vi "HEWH Find Vn.vi"(8 "error in (no error)":errorcluster, 11 "UEF Calculated Values Input":T1 {"Data Indexes"."15 sec after Draw Index" format="%#.2f"; "Data Indexes"."15 sec after Draw Timestamp" format="%#.2f"; "Data Indexes"."Test Start Timestamp" format="%.2f"; "Data Indexes"."Test End Timestamp" format="%.2f"; "Data Indexes"."T0 Timestamp" format="%.2f"; "Data Indexes"."Tsf Timestamp" format="%.2f"; "Data Indexes"."Tsu0 Timestamp" format="%.2f"; "Data Indexes"."Tmax1 Timestamp" format="%.2f"; "Data Indexes"."Draw Index Timestamp" format="%#.2f"; "Data Indexes"."Non-Draw Timestamp" format="%#.2f"; "Data Indexes"."Heating Timestamp" format="%#.2f"; "Data Indexes"."Start Energy (BTU-Gas)" format="%.6f"; "Data Indexes"."Start Watt Hours" format="%.6f"; "Static Data"."V - Volume of Wh (True)" format="%.5f"; "Static Data"."T-Ambinet Nominal (°F)" format="%.5f"; "Static Data"."T-Inlet Setpoint (°F)" format="%.5f"; "Static Data"."T-Wh Setpoint (°F)" format="%.5f"; "Sampled Data"."Qe (Wh)" format="%.5f"; "Sampled Data"."Tau stby2 (hr)" format="%.5f"; "Sampled Data"."Tastby2 (°F)" format="%.5f"; "Sampled Data"."Qf (BTU)" format="%.5f"; "Sampled Data"."Qe (BTU)" format="%.5f"; "Sampled Data"."Tmax1 (°F)" format="%.5f"; "Sampled Data"."T0 (°F)" format="%.5f"; "Sampled Data"."Qr (BTU)" format="%.5f"; "Sampled Data"."T 24(°F)" format="%.5f"; "Sampled Data"."T astby(°F)" format="%.5f"; "Sampled Data"."T tstby(°F)" format="%.5f"; "Sampled Data"."T su0(°F)" format="%.5f"; "Sampled Data"."T suf(°F)" format="%.5f"; "Sampled Data"."Tau stby_1 (hr)" format="%.5f"; "Sampled Data"."Qsuf (BTU)" format="%.5f"; "Sampled Data"."Qsu0 (BTU)" format="%.5f"; "Calculated Values"."Draw Bonus Volume (gal)" format="%.6f"; "Calculated Values"."Adjustment Factor" format="%.6f"; "Calculated Values"."T*avg_del(n-1)" format="%.6f"; "Calculated Values"."T*min(n-1)" format="%.6f"; "Calculated Values"."T*avg_del(n)" format="%.6f"; "Calculated Values"."Vn" format="%.6f"; "Calculated Values"."Qdm (BTU)" format="%.6f"; "Calculated Values"."QHWD (BTU)" format="%.6f"; "Calculated Values"."QHW (BTU)" format="%.6f"; "Calculated Values"."UEF" format="%.6f"; "Calculated Values"."QHW67 (BTU)" format="%.6f"; "Calculated Values"."Qda (BTU)" format="%.6f"; "Calculated Values"."Qd (BTU)" format="%.6f"; "Calculated Values"."Q (BTU)" format="%.6f"; "Calculated Values"."UA (BTU/(hr*F))" format="%.6f"; "Calculated Values"."Qhr (BTU/hr)" format="%.6f"; "Calculated Values"."Qstby (BTU)" format="%.6f"; "Calculated Values"."nu_r" format="%.6f"; "Calculated Values"."CpUEF (BTU/(lb*F))" format="%.6f"; "Calculated Values"."rho_nu (lb/gal)" format="%.6f"; "Calculated Values"."V1- Vol (Gal)" format="%.6f"; "Calculated Values"."M cluster mass removed (lb)" format="%.6f"; "Calculated Values"."Cp theoretical (BTU/(lbm °F))" format="%.6f"; "Calculated Values"."Tin1 - Mean Inlet 1st Cluster (°F)" format="%.6f"; "Calculated Values"."Tdel1-Mean Outlet 1st Cluster(°F)" format="%.6f"; "Calculated Values"."Cp 24 (BTU/(lb*F))" format="%.6f"; "Calculated Values"."Cp standby (BTU/(lb*F))" format="%.6f"; "Calculated Values"."Cp2 (BTU/(lb*F))" format="%.6f"; "Calculated Values"."Cp1 (BTU/(lb*F))" format="%.6f"; "Calculated Values"."rho 24 (lb/gal)" format="%.6f"; "Calculated Values"."rho standby (lb/gal)" format="%.6f"; "Calculated Values"."rho 2 (lb/gal)" format="%.6f"; "Calculated Values"."Density of cold water All (lbm/gal)" format="%#.3g"; "Calculated Values"."CpHW (BTU/(lbm °F))" format="%#.3g"; "Calculated Values"."Density of hot water All (lbm/gal)" format="%#.3g"; "Calculated Values"."Mass of water All (lbm)" format="%#.3f"}) -> (0 "error out":errorcluster, 3 "UEF Calculated Values Output":T1 {"Data Indexes"."15 sec after Draw Index" format="%#.2f"; "Data Indexes"."15 sec after Draw Timestamp" format="%#.2f"; "Data Indexes"."Test Start Timestamp" format="%.2f"; "Data Indexes"."Test End Timestamp" format="%.2f"; "Data Indexes"."T0 Timestamp" format="%.2f"; "Data Indexes"."Tsf Timestamp" format="%.2f"; "Data Indexes"."Tsu0 Timestamp" format="%.2f"; "Data Indexes"."Tmax1 Timestamp" format="%.2f"; "Data Indexes"."Draw Index Timestamp" format="%#.2f"; "Data Indexes"."Non-Draw Timestamp" format="%#.2f"; "Data Indexes"."Heating Timestamp" format="%#.2f"; "Data Indexes"."Start Energy (BTU-Gas)" format="%.6f"; "Data Indexes"."Start Watt Hours" format="%.6f"; "Static Data"."V - Volume of Wh (True)" format="%.5f"; "Static Data"."T-Ambinet Nominal (°F)" format="%.5f"; "Static Data"."T-Inlet Setpoint (°F)" format="%.5f"; "Static Data"."T-Wh Setpoint (°F)" format="%.5f"; "Sampled Data"."Qe (Wh)" format="%.5f"; "Sampled Data"."Tau stby2 (hr)" format="%.5f"; "Sampled Data"."Tastby2 (°F)" format="%.5f"; "Sampled Data"."Qf (BTU)" format="%.5f"; "Sampled Data"."Qe (BTU)" format="%.5f"; "Sampled Data"."Tmax1 (°F)" format="%.5f"; "Sampled Data"."T0 (°F)" format="%.5f"; "Sampled Data"."Qr (BTU)" format="%.5f"; "Sampled Data"."T 24(°F)" format="%.5f"; "Sampled Data"."T astby(°F)" format="%.5f"; "Sampled Data"."T tstby(°F)" format="%.5f"; "Sampled Data"."T su0(°F)" format="%.5f"; "Sampled Data"."T suf(°F)" format="%.5f"; "Sampled Data"."Tau stby_1 (hr)" format="%.5f"; "Sampled Data"."Qsuf (BTU)" format="%.5f"; "Sampled Data"."Qsu0 (BTU)" format="%.5f"; "Calculated Values"."Draw Bonus Volume (gal)" format="%.6f"; "Calculated Values"."Adjustment Factor" format="%.6f"; "Calculated Values"."T*avg_del(n-1)" format="%.6f"; "Calculated Values"."T*min(n-1)" format="%.6f"; "Calculated Values"."T*avg_del(n)" format="%.6f"; "Calculated Values"."Vn" format="%.6f"; "Calculated Values"."Qdm (BTU)" format="%.6f"; "Calculated Values"."QHWD (BTU)" format="%.6f"; "Calculated Values"."QHW (BTU)" format="%.6f"; "Calculated Values"."UEF" format="%.6f"; "Calculated Values"."QHW67 (BTU)" format="%.6f"; "Calculated Values"."Qda (BTU)" format="%.6f"; "Calculated Values"."Qd (BTU)" format="%.6f"; "Calculated Values"."Q (BTU)" format="%.6f"; "Calculated Values"."UA (BTU/(hr*F))" format="%.6f"; "Calculated Values"."Qhr (BTU/hr)" format="%.6f"; "Calculated Values"."Qstby (BTU)" format="%.6f"; "Calculated Values"."nu_r" format="%.6f"; "Calculated Values"."CpUEF (BTU/(lb*F))" format="%.6f"; "Calculated Values"."rho_nu (lb/gal)" format="%.6f"; "Calculated Values"."V1- Vol (Gal)" format="%.6f"; "Calculated Values"."M cluster mass removed (lb)" format="%.6f"; "Calculated Values"."Cp theoretical (BTU/(lbm °F))" format="%.6f"; "Calculated Values"."Tin1 - Mean Inlet 1st Cluster (°F)" format="%.6f"; "Calculated Values"."Tdel1-Mean Outlet 1st Cluster(°F)" format="%.6f"; "Calculated Values"."Cp 24 (BTU/(lb*F))" format="%.6f"; "Calculated Values"."Cp standby (BTU/(lb*F))" format="%.6f"; "Calculated Values"."Cp2 (BTU/(lb*F))" format="%.6f"; "Calculated Values"."Cp1 (BTU/(lb*F))" format="%.6f"; "Calculated Values"."rho 24 (lb/gal)" format="%.6f"; "Calculated Values"."rho standby (lb/gal)" format="%.6f"; "Calculated Values"."rho 2 (lb/gal)" format="%.6f"; "Calculated Values"."Density of cold water All (lbm/gal)" format="%#.3g"; "Calculated Values"."CpHW (BTU/(lbm °F))" format="%#.3g"; "Calculated Values"."Density of hot water All (lbm/gal)" format="%#.3g"; "Calculated Values"."Mass of water All (lbm)" format="%#.3f"})   [LabVIEW 2023]
uses:
  Type Definitions/UEF Constants.ctl
  Type Definitions/HEWH Draw Stats.ctl
  Type Definitions/HEWH FHR Draw Type.ctl
  Type Definitions/FHR Bins.ctl
  Type Definitions/HEWH Meter Type.ctl
panel:
  # "FHR"
  # "FHR"
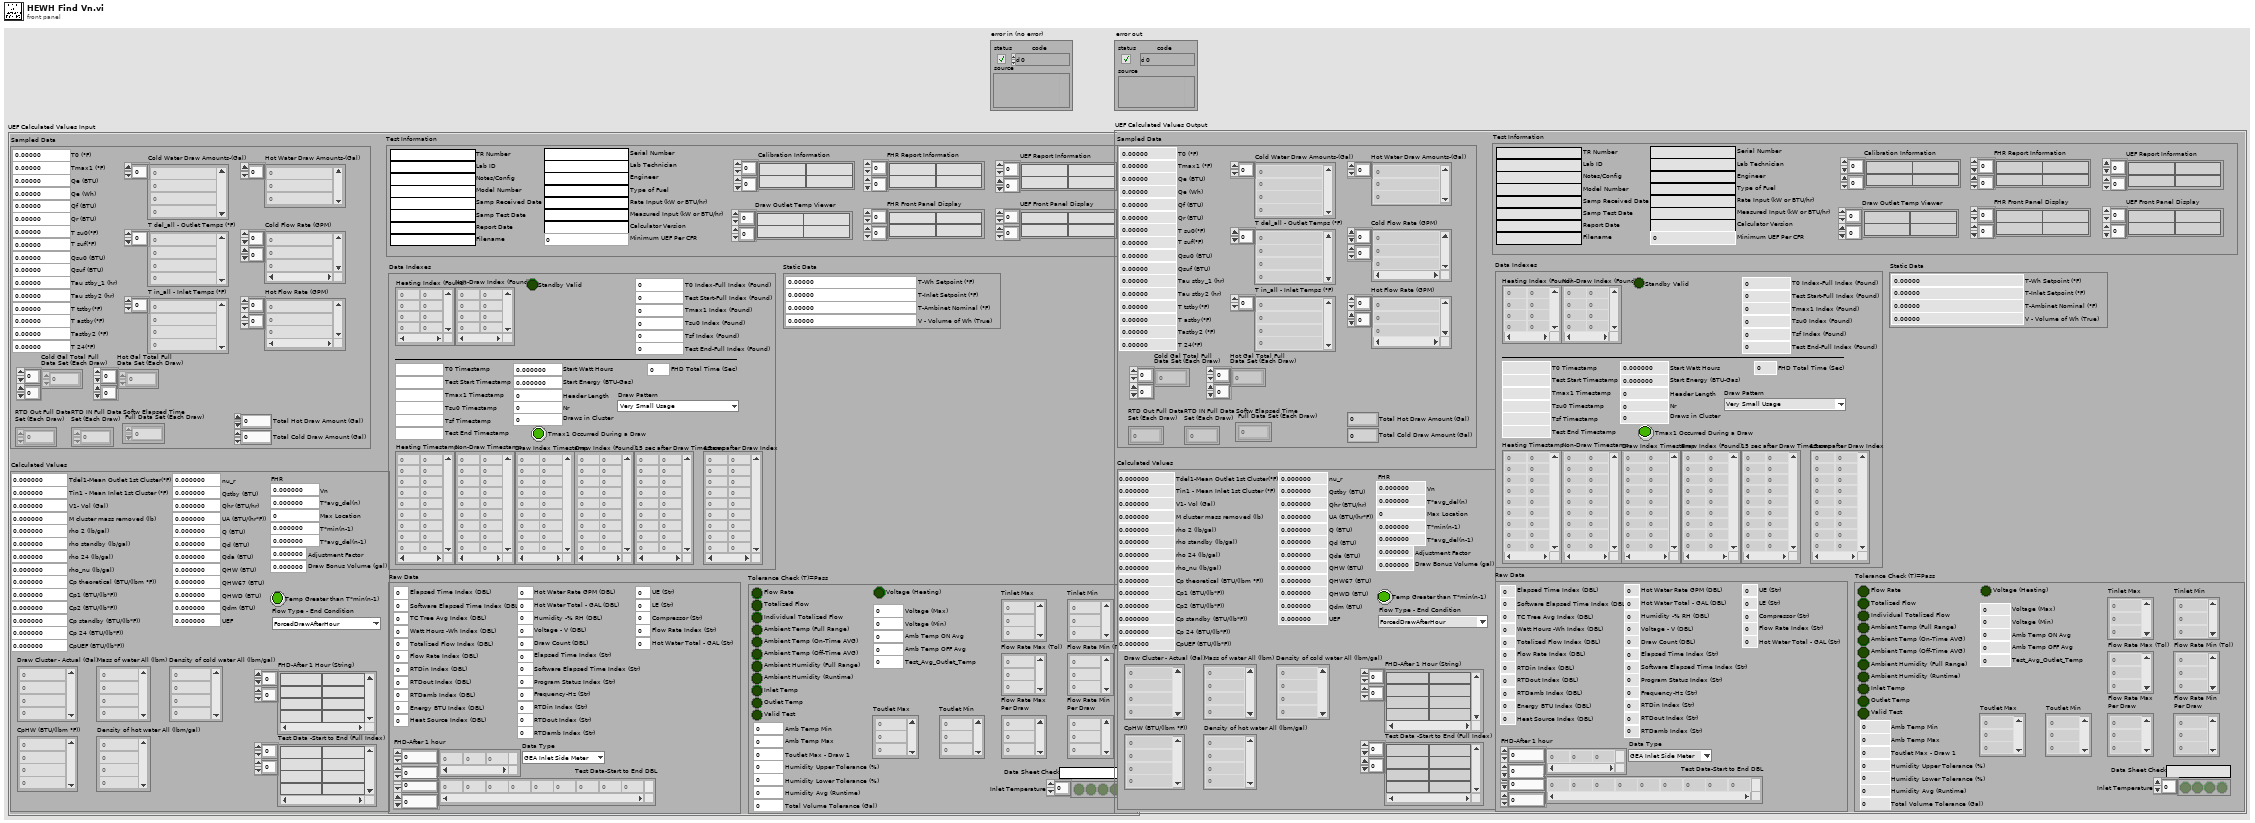
[diagram p1: front panel]
types:
  T1 = typedef "UEF Constants.ctl" = cluster{"Calculated Values":T2, "Sampled Data":cluster{"Cold Water Draw Amounts-(Gal)":dbl[], "T del_all - Outlet Temps (°F)":dbl[], "T in_all - Inlet Temps (°F)":dbl[], "Qsu0 (BTU)":dbl, "Qsuf (BTU)":dbl, "Tau stby_1 (hr)":dbl, "T suf(°F)":dbl, "T su0(°F)":dbl, "T tstby(°F)":dbl, "T astby(°F)":dbl, "T 24(°F)":dbl, "Qr (BTU)":dbl, "T0 (°F)":dbl, "Tmax1 (°F)":dbl, "Qe (BTU)":dbl, "Qf (BTU)":dbl, "Tastby2 (°F)":dbl, "RTD Out Full Data\nSet (Each Draw)":dbl[][], "RTD IN Full Data\nSet (Each Draw)":dbl[][], "Tau stby2 (hr)":dbl, "Hot Water Draw Amounts-(Gal)":dbl[], "Cold Flow Rate (GPM)":dbl[][], "Hot Flow Rate (GPM)":dbl[][], "Softw Elapsed Time\n Full Data Set (Each Draw)":dbl[][], "Cold Gal Total Full\nData Set (Each Draw)":dbl[][], "Total Hot Draw Amount (Gal) ":dbl, "Total Cold Draw Amount (Gal)":dbl, "Qe (Wh)":dbl, "Hot Gal Total Full\nData Set (Each Draw)":dbl[][]}, "Static Data":cluster{"T-Wh Setpoint (°F)":dbl, "T-Inlet Setpoint (°F)":dbl, "T-Ambinet Nominal (°F)":dbl, "V - Volume of Wh (True)":dbl}, "Data Indexes":cluster{"Test Start-Full Index (Found)":i32, "Header Length":i32, "Draw Index (Found)":i32[][], "Nr":i32, "Start Watt Hours":dbl, "Tsu0 Index (Found)":i32, "Tsf Index (Found)":i32, "Start Energy (BTU-Gas)":dbl, "Draws in Cluster":i32, "T0 Index-Full Index (Found)":i32, "Non-Draw Index (Found)":i32[][], "Tmax1 Index (Found)":i32, "Test End-Full Index (Found)":i32, "Heating Index (Found)":i32[][], "Heating Timestamp":dbl[][], "Non-Draw Timestamp":dbl[][], "Draw Index Timestamp":dbl[][], "Tmax1 Timestamp":dbl, "Tsu0 Timestamp":dbl, "Tsf Timestamp":dbl, "T0 Timestamp":dbl, "Test End Timestamp":dbl, "Test Start Timestamp":dbl, "15 sec after Draw Timestamp":dbl[][], "15 sec after Draw Index":dbl[][], "Tmax1 Occurred During a Draw":bool, "FHD Total Time (Sec)":dbl, "Draw Pattern":T4, "Standby Valid":bool}, "Raw Data":cluster{"Elapsed Time Index (DBL)":i32, "Software Elapsed Time Index (DBL)":i32, "TC Tree Avg Index (DBL)":i32, "Watt Hours -Wh Index (DBL)":i32, "Energy BTU Index (DBL)":i32, "Totalized Flow Index (DBL)":i32, "Flow Rate Index (DBL)":i32, "Program Status Index (Str)":i32, "RTDin Index (DBL)":i32, "RTDout Index (DBL)":i32, "RTDamb Index (DBL)":i32, "Test Data-Start to End DBL":dbl[][], "Data Type":T5, "Heat Source Index (DBL)":i32, "Hot Water Rate GPM (DBL)":i32, "Hot Water Total - GAL (DBL)":i32, "FHD-After 1 hour":dbl[][], "Humidity -% RH (DBL)":i32, "Voltage - V (DBL)":i32, "Draw Count (DBL)":i32, "Elapsed Time Index (Str)":i32, "Software Elapsed Time Index (Str)":i32, "Frequency-Hz (Str)":i32, "RTDin Index (Str)":i32, "RTDout Index (Str)":i32, "RTDamb Index (Str)":i32, "UE (Str)":i32, "LE (Str)":i32, "Compressor (Str)":i32, "Flow Rate Index (Str)":i32, "Hot Water Total - GAL (Str)":i32}, "Tolerance Check (T)=Pass":cluster{"Flow Rate":bool, "Totalized Flow":bool, "Ambient Temp (Full Range)":bool, "Ambient Humidity (Full Range)":bool, "Inlet Temp":bool, "Outlet Temp":bool, "Valid Test":bool, "Individual Totalized Flow":bool, "Data Sheet Check":string, "Inlet Temperature":bool[], "Tinlet Max":dbl[], "Tinlet Min":dbl[], "Flow Rate Max (Tol)":dbl[], "Flow Rate Min (Tol)":dbl[], "Amb Temp Max":dbl, "Amb Temp Min":dbl, "Toutlet Max - Draw 1":dbl, "Humidity Upper Tolerance (%)":dbl, "Total Volume Tolerance (Gal)":dbl, "Humidity Lower Tolerance (%)":dbl, "Flow Rate Max\nPer Draw":dbl[], "Flow Rate Min\nPer Draw":dbl[], "Ambient Humidity (Runtime)":bool, "Humidity Avg (Runtime)":dbl, "Ambient Temp (On-Time AVG)":bool, "Ambient Temp (Off-Time AVG)":bool, "Amb Temp OFF Avg":dbl, "Amb Temp ON Avg":dbl, "Voltage (Heating)":bool, "Voltage (Min)":dbl, "Voltage (Max)":dbl, "Toutlet Max":dbl[], "Toutlet Min":dbl[], "Test_Avg_Outlet_Temp":dbl}, "Test Information":cluster{"TR Number":string, "Lab ID":string, "Notes/Config":string, "Model Number":string, "Serial Number":string, "Lab Technician":string, "Engineer":string, "Type of Fuel":string, "Samp Received Date":string, "Samp Test Date":string, "Report Date":string, "Rate Input (kW or BTU/hr)":string, "Measured Input (kW or BTU/hr)":string, "Filename":string, "Calibration Information":string[][], "Calculator Version":string, "Minimum UEF Per CFR":dbl, "UEF Report Information":string[][], "FHR Report Information":string[][], "FHR Front Panel Display":string[][], "UEF Front Panel Display":string[][], "Draw Outlet Temp Viewer":string[][]}}
  T2 = typedef "HEWH Draw Stats.ctl" = cluster{"Draw Cluster - Actual (Gal)":dbl[], "Mass of water All (lbm)":dbl[], "Density of hot water All (lbm/gal)":dbl[], "CpHW (BTU/(lbm °F))":dbl[], "rho 2 (lb/gal)":dbl, "rho standby (lb/gal)":dbl, "rho 24 (lb/gal)":dbl, "Cp1 (BTU/(lb*F))":dbl, "Cp2 (BTU/(lb*F))":dbl, "Cp standby (BTU/(lb*F))":dbl, "Cp 24 (BTU/(lb*F))":dbl, "nu_r":dbl, "Qstby (BTU)":dbl, "Qhr (BTU/hr)":dbl, "UA (BTU/(hr*F))":dbl, "Q (BTU)":dbl, "Qd (BTU)":dbl, "Qda (BTU)":dbl, "QHW67 (BTU)":dbl, "UEF":dbl, "Tdel1-Mean Outlet 1st Cluster(°F)":dbl, "Tin1 - Mean Inlet 1st Cluster (°F)":dbl, "Cp theoretical (BTU/(lbm °F))":dbl, "M cluster mass removed (lb)":dbl, "V1- Vol (Gal)":dbl, "Test Data -Start to End (Full Index)":string[][], "rho_nu (lb/gal)":dbl, "Density of cold water All (lbm/gal)":dbl[], "CpUEF (BTU/(lb*F))":dbl, "QHW (BTU)":dbl, "QHWD (BTU)":dbl, "Qdm (BTU)":dbl, "FHD-After 1 Hour (String)":string[][], "Vn":dbl, "T*avg_del(n)":dbl, "Max Location":i32, "T*min(n-1)":dbl, "T*avg_del(n-1)":dbl, "Temp Greater than T*min(n-1)":bool, "Adjustment Factor":dbl, "Draw Bonus Volume (gal)":dbl, "Flow Type - End Condition":T3}
  T3 = typedef "HEWH FHR Draw Type.ctl" = enum16{"ForcedDrawAfterHour", "HeatingCutoffBeforeHour"}
  T4 = typedef "FHR Bins.ctl" = enum16{"Very Small Usage", "Low Usage", "Medium Usage", "High Usage", "Undefined"}
  T5 = typedef "HEWH Meter Type.ctl" = enum16{"GEA Inlet Side Meter", "GEA Outlet Side Meter", "CSA Inlet Side Meter"}
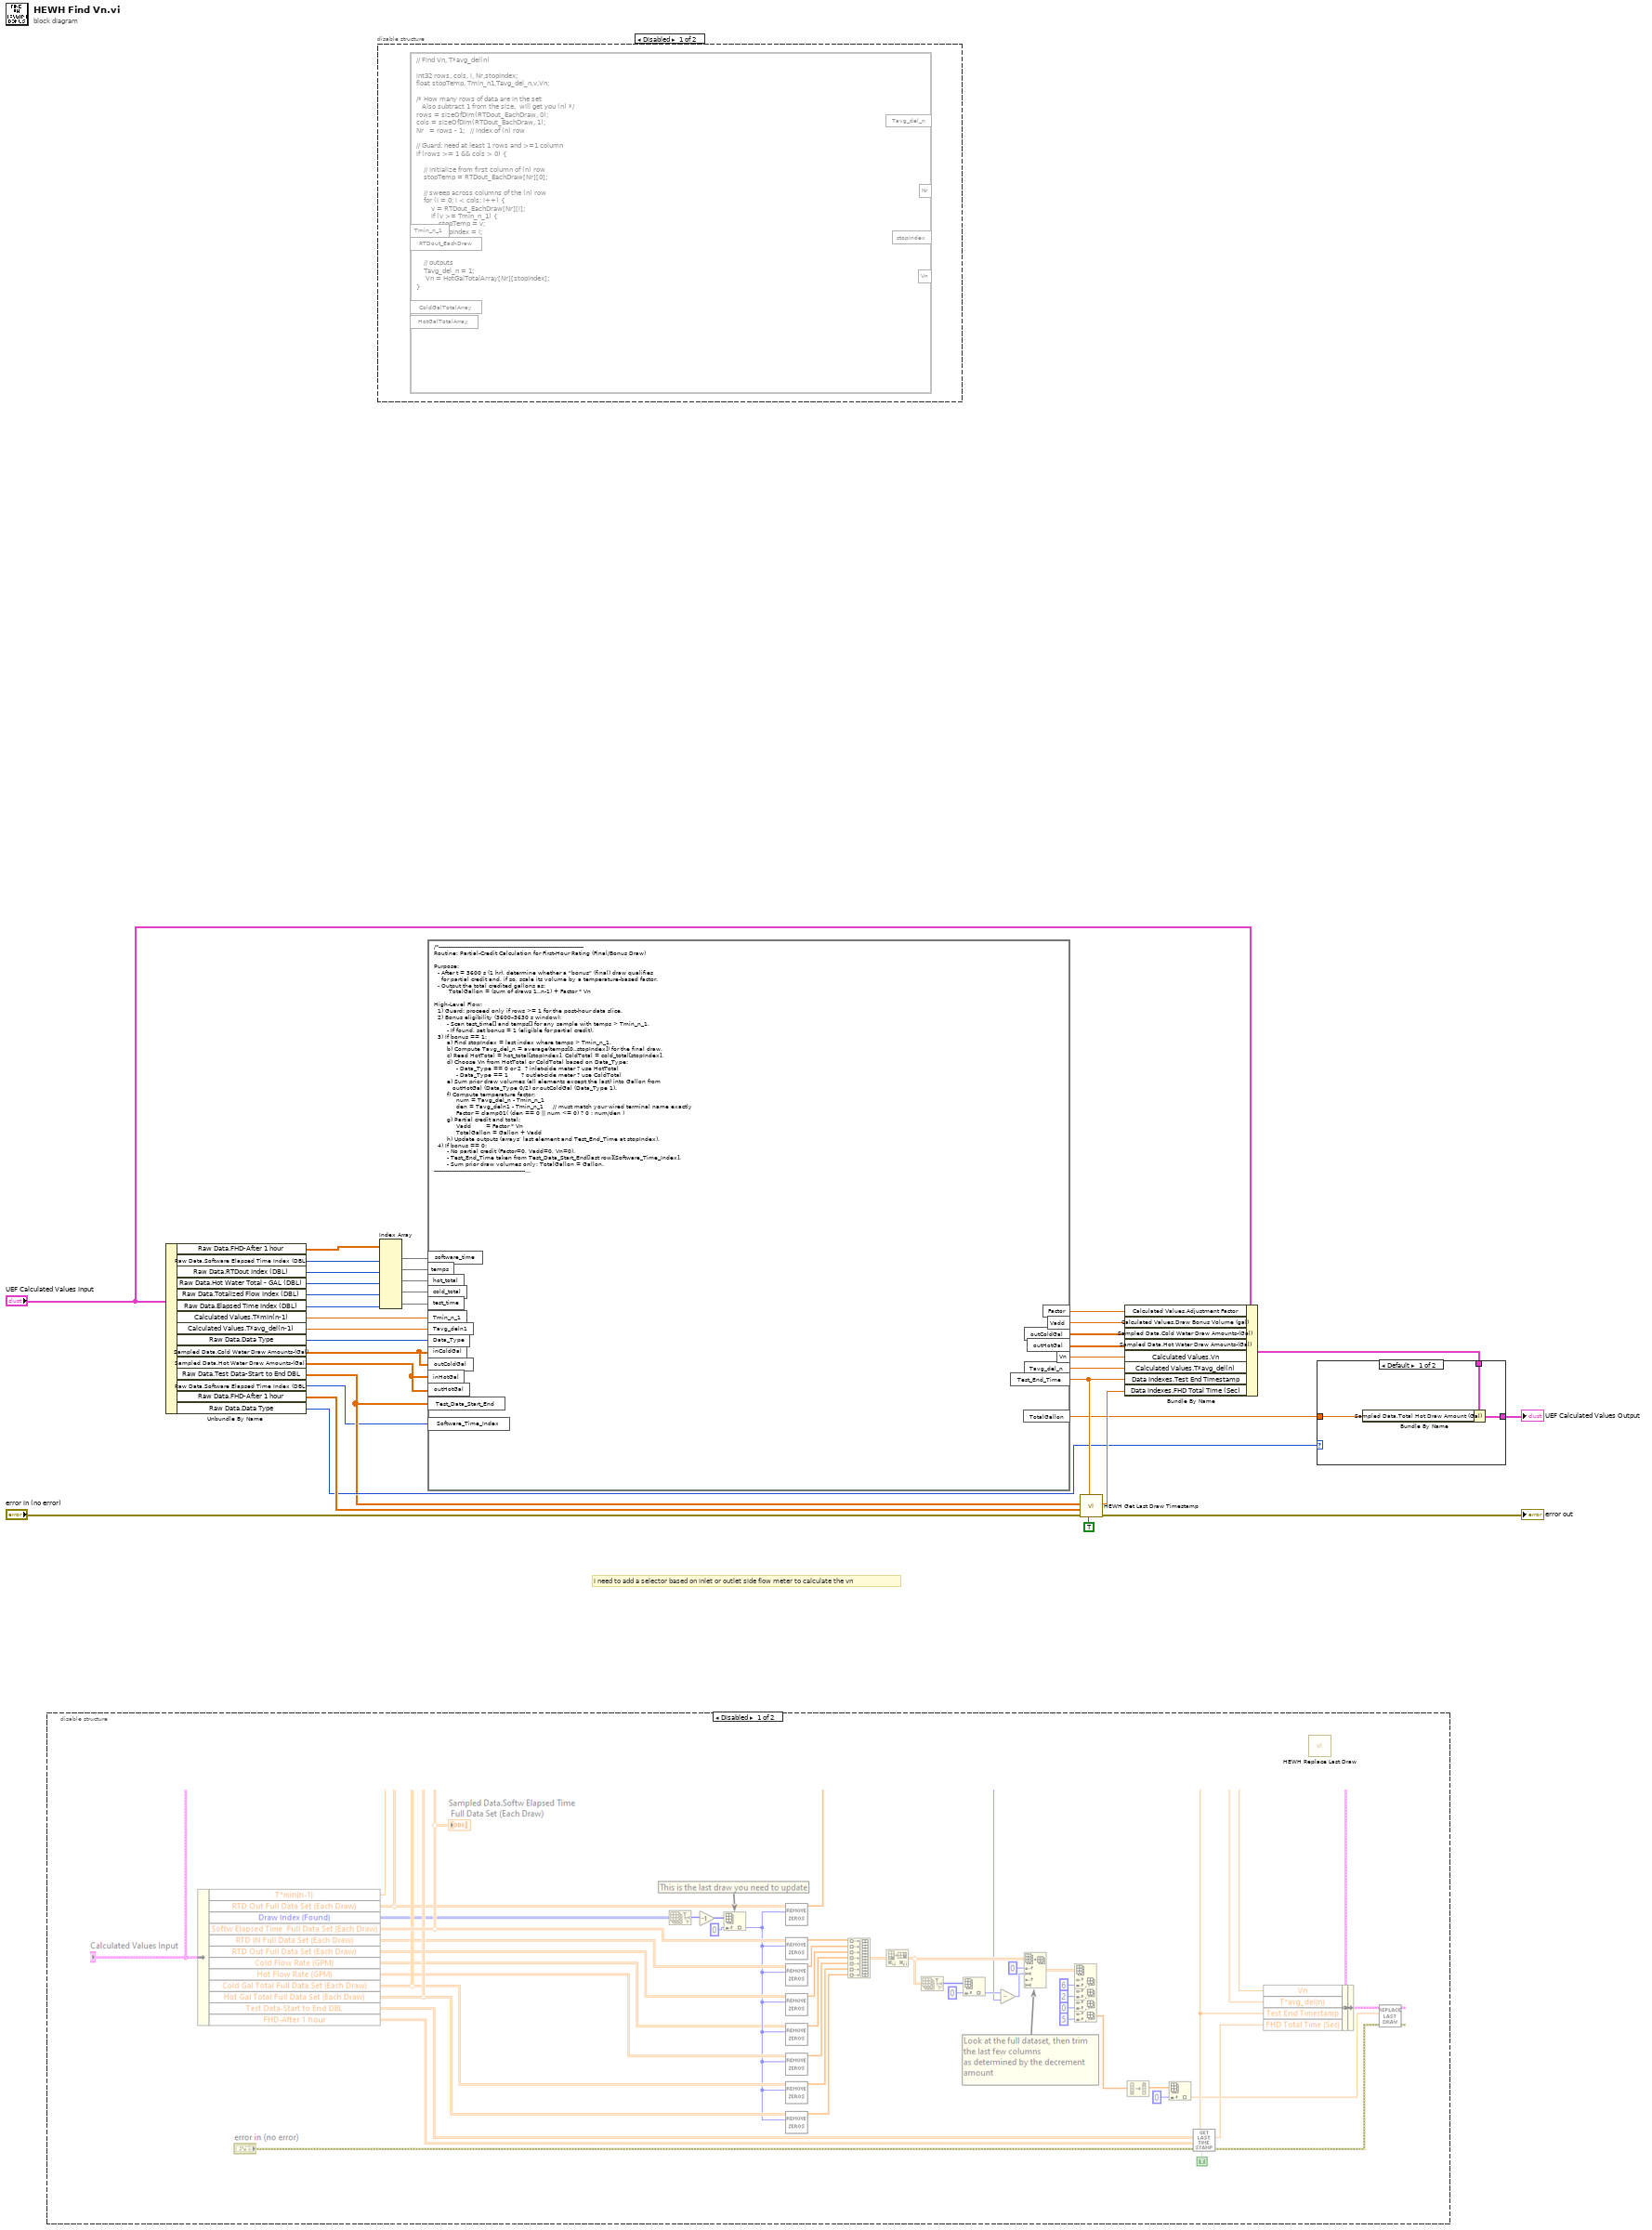
[diagram p0: block diagram]
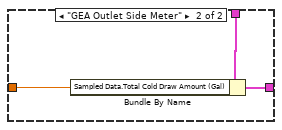
[diagram p2: hidden frame]
diagram:
  # "i need to add a selector based on inlet or outlet side flow meter to calculate the vn"
  n1 = disable-structure shown="Disabled" {
    frame Disabled {
      n2 = call "HEWH Replace Last Draw.vi"() -> ()  [unwired: 10 in, 2 out]
    }
    frame Enabled {
    }
  }
  n3 = Unbundle By Name("UEF Calculated Values Input") -> ("Raw Data.FHD-After 1 hour"=w21:dbl[][], "Raw Data.Software Elapsed Time Index (DBL)"=w20:i32, "Raw Data.RTDout Index (DBL)"=w19:i32, "Raw Data.Hot Water Total - GAL (DBL)"=w16:i32, "Raw Data.Totalized Flow Index (DBL)"=w15:i32, "Raw Data.Elapsed Time Index (DBL)"=w11:i32, "Calculated Values.T*min(n-1)"=w30:dbl, "Calculated Values.T*avg_del(n-1)"=w9:dbl, "Raw Data.Data Type"=w10:T5, "Sampled Data.Cold Water Draw Amounts-(Gal)"=w26:dbl[], "Sampled Data.Hot Water Draw Amounts-(Gal)"=w25:dbl[], "Raw Data.Test Data-Start to End DBL"=w2:dbl[][], "Raw Data.Software Elapsed Time Index (DBL)"=w1:i32, "Raw Data.FHD-After 1 hour"=w34:dbl[][], "Raw Data.Data Type"=w4:T5)
  n4 = disable-structure shown="Disabled" {
    frame Disabled {
      n5 = formula code="// Find Vn, T*avg_del(n)\n\nint32 rows, cols, i, Nr,stopIndex;\nfloat stopTemp, Tmin_n1,Tavg_del_n,v,Vn;\n\n/* How many rows of data are in the set\n   Also subtract 1 from the size,  will get you (n) */\nrows = sizeOfDim(RTDout_EachDraw, 0);\ncols = sizeOfDim(RTDout_EachDraw, 1);\nNr   = rows - 1;   // index of (n) row\n\n// Guard: need at least 1 rows and >=1 column\nif (rows >= 1 && cols > 0) {\n\n    // initialize from first column of (n) row\n    stopTemp = RTDout_EachDraw[Nr][0];\n\n    // sweep across columns of the (n) row\n    for (i = 0; i < cols; i++) {\n        v = RTDout_EachDraw[Nr][i];\n        if (v >= Tmin_n_1) {\n            stopTemp = v;\n            stopIndex = i;\n        }\n    }\n\n    // outputs\n    Tavg_del_n = 1;\n     Vn = HotGalTotalArray[Nr][stopIndex];\n}"() -> ()  [unwired: 4 in, 4 out]
    }
    frame Enabled {
    }
  }
  n6 = Index Array "Index Array"(array=w21, index (col) #1=w20, index (col) #2=w19, index (col) #3=w16, index (col) #4=w15, index (col) #5=w11) -> (element #1=w18:dbl[], element #2=w17:dbl[], element #3=w14:dbl[], element #4=w13:dbl[], element #5=w12:dbl[])  [unwired: 5 in]
  n7 = formula code="/*------------------------------------------------------------------------------\nRoutine: Partial-Credit Calculation for First-Hour Rating (Final/Bonus Draw)\n\nPurpose:\n  - After t = 3600 s (1 hr), determine whether a \"bonus\" (final) draw qualifies\n    for partial credit and, if so, scale its volume by a temperature-based factor.\n  - Output the total credited gallons as:\n        TotalGallon = (sum of draws 1..n-1) + Factor * Vn\n\nHigh-Level Flow:\n  1) Guard: proceed only if rows >= 1 for the post-hour data slice.\n  2) Bonus eligibility (3600–3630 s window):\n       - Scan test_time[] and temps[] for any sample with temps > Tmin_n_1.\n       - If found, set bonus = 1 (eligible for partial credit).\n  3) If bonus == 1:\n       a) Find stopIndex = last index where temps > Tmin_n_1.\n       b) Compute Tavg_del_n = average(temps[0..stopIndex]) for the final draw.\n       c) Read HotTotal = hot_total[stopIndex], ColdTotal = cold_total[stopIndex].\n       d) Choose Vn from HotTotal or ColdTotal based on Data_Type:\n            - Data_Type == 0 or 2  ? inlet-side meter ? use HotTotal\n            - Data_Type == 1       ? outlet-side meter ? use ColdTotal\n       e) Sum prior draw volumes (all elements except the last) into Gallon from\n          outHotGal (Data_Type 0/2) or outColdGal (Data_Type 1).\n       f) Compute temperature factor:\n            num = Tavg_del_n - Tmin_n_1\n            den = Tavg_deln1 - Tmin_n_1     // must match your wired terminal name exactly\n            Factor = clamp01( (den == 0 || num <= 0) ? 0 : num/den )\n       g) Partial credit and total:\n            Vadd        = Factor * Vn\n            TotalGallon = Gallon + Vadd\n       h) Update outputs (arrays’ last element and Test_End_Time at stopIndex).\n  4) If bonus == 0:\n       - No partial credit (Factor=0, Vadd=0, Vn=0).\n       - Test_End_Time taken from Test_Data_Start_End[last row][Software_Time_Index].\n       - Sum prior draw volumes only; TotalGallon = Gallon.\n------------------------------------------------------------------------------*/\n\n\nint32 rows, i, Nr, stopIndex, count,nCold, nHot,lenVol,idx,Full_Data_Rows;\nfloat stopTemp, Tavg_del_n, v, Vn,ColdTotal,HotTotal,num,den;\nfloat sumV, avgV,t;\nfloat Gallon = 0.0;                 // Total gallons\nint32 bonus    = 0;   // 0 = false, 1 = true\nint32 hitIndex = -1;  // index of first qualifying sample\n\n/* How many rows of data are in the set\n   Also subtract 1 from the size, will get you (n) */\nrows = sizeOfDim(temps, 0);    // Get the number of rows in the array, this is the 0\nNr   = rows - 1;   // index of (n) row\n\n// Guard: need at least 1 row\nif (rows >= 1) {\n\n//-----------------------------------------------------------------------------------------------\n//-- Check if there is a bonus draw\n   for (i = 0; i <= Nr; i++) {\n     t = test_time[i];\n     v = temps[i];\n  \n     // Ensure sample is within 3600–3630 s window\n     if (t >= 3600.0 && t <= 3630.0) {\n       if (v == v) {               // skip NaN\n         if (v > Tmin_n_1) {          // CFR: strictly greater than T*min,n-1\n           bonus    = 1;\n           hitIndex = i;\n           break;\n         }\n       }\n     }\n   }\n\n//-----------------------------------------------------------------------------------------------\n\n// Check if Bonus Draw Logic Should Apply\nif (bonus == 1) {\n\n    // initialize from first column of (n) row\n    stopTemp  = 0;\n    stopIndex = 0;                  // safe default\n// -----------------------------------------------------------------------------------------------\n    // sweep across rows of the (n) row to locate stop point, you will do this for the full array\n    for (i = 0; i <= Nr; i++) {\n        v = temps[i];\n        if (v > Tmin_n_1) {        // last index where threshold met\n            stopTemp  = v;\n            stopIndex = i;\n        }\n    }\n// -----------------------------------------------------------------------------------------------\n    // ---- average v from i = 0 to i = stopIndex (inclusive) ----\n    sumV  = 0.0;\n    count = 0;\n// -----------------------------------------------------------------------------------------------\n    for (i = 0; i <= stopIndex; i++) {\n        sumV += temps[i];\n        count += 1;\n    }\n// -----------------------------------------------------------------------------------------------\n    if (count > 0) {\n        avgV = sumV / count;\n       } \n    else {\n        avgV = 0.0;                 // safety fallback\n    }\n// -----------------------------------------------------------------------------------------------\n\n    // outputs\n    Tavg_del_n = avgV;                                             // average outlet temperature of draw (n) up to stop index\n    HotTotal = hot_total[stopIndex];                      // Hot gallons at stop index\n    ColdTotal = cold_total[stopIndex];                   // Cold gallons at stop index\n    Test_End_Time = software_time[stopIndex];   // Software elapsed time at stop index\n\n//-----------------------------------------------------------------------------------------------\n/* Cold, Update the array and replace the element with the stop index draw amount */\nnCold = sizeOfDim(inColdGal, 0);\n//-----------------------------------------------------------------------------------------------\nfor (i = 0; i < nCold; i++) {\n    outColdGal[i] = inColdGal[i];\n}\n//-----------------------------------------------------------------------------------------------\nif (nCold > 0) {\n    outColdGal[nCold - 1] = ColdTotal;\n}\n//-----------------------------------------------------------------------------------------------\n/* Hot, Update the array and replace the element with the stop index draw amount */\nnHot = sizeOfDim(inHotGal, 0);\n//-----------------------------------------------------------------------------------------------\nfor (i = 0; i < nHot; i++) {\n    outHotGal[i] = inHotGal[i];\n}\n//-----------------------------------------------------------------------------------------------\nif (nHot > 0) {\n    outHotGal[nHot - 1] = HotTotal;\n}\n//-----------------------------------------------------------------------------------------------\n// If Data Type = 0 (GEA Inlet Side) or 2 (CSA Inlet Side), than this means the flow meter is on the inlet side\nif (Data_Type == 0 || Data_Type == 2) {\n\n   // Find the length of the volume array\n   lenVol = sizeOfDim(outHotGal, 0);\n//-----------------------------------------------------------------------------------------------\n   /* sum all elements except the last one */\n   if (lenVol > 1) {\n       for (idx = 0; idx < lenVol - 1; idx++) {\n           Gallon += outHotGal[idx];\n       }\n   }\n//-----------------------------------------------------------------------------------------------\n   Vn = HotTotal;\n}\n//-----------------------------------------------------------------------------------------------\n\n// This is the case where the flow meter is on the outlet side of the water heater\nelse if (Data_Type == 1) {\n\n   // Find the length of the volume array\n   lenVol = sizeOfDim(outColdGal, 0);\n//-----------------------------------------------------------------------------------------------\n   /* sum all elements except the last one */\n   if (lenVol > 1) {\n       for (idx = 0; idx < lenVol - 1; idx++) {\n           Gallon += outColdGal[idx];\n       }\n   }\n//-----------------------------------------------------------------------------------------------\n   Vn = ColdTotal;\n}\n//-----------------------------------------------------------------------------------------------\n// Step 1: Calculate Temperature Factor (robust + clamped [0,1])\n\n       num = Tavg_del_n - Tmin_n_1;     // numerator\n       den = Tavg_deln1 - Tmin_n_1;     // denominator\n\nif (den == 0.0) {\n    Factor = 0.0;                       // avoid divide-by-zero\n}\nelse if (num <= 0.0) {\n    Factor = 0.0;                       // Negative factors lead to subtracting volume, so make the factor 0 in this case.\n}\nelse {\n    Factor = num / den;                 // compute raw factor\n\n    // Clamp to [0, 1]\n    if (Factor < 0.0) {\n        Factor = 0.0;\n    } else if (Factor > 1.0) {\n        Factor = 1.0;\n    }\n}\n//-----------------------------------------------------------------------------------------------\n    // Step 2: Calculate Adjusted Volume for Final Draw\n    Vadd = Factor * Vn;\n\n    // Step 3: Calculate Total Gallons\n    TotalGallon = Gallon + Vadd;\n//-----------------------------------------------------------------------------------------------\n}\n// If bonus ==0, then do the below.\nelse {\n    Full_Data_Rows = sizeOfDim(Test_Data_Start_End, 0)-1;    // Get the number of rows in the array\n\n    // No bonus draw applied; keep values unchanged\n    Factor               = 0.0;\n    Vadd                 = 0.0;\n    Tavg_del_n       = 0.0;\n    Test_End_Time = Test_Data_Start_End[Full_Data_Rows][Software_Time_Index];   // If no bonus draw, its just the last time\n    Vn                      = 0.0;\n\n    //-----------------------------------------------------------------------------------------------\n    // If Data Type = 0 (GEA Inlet Side) or 2 (CSA Inlet Side), than this means the flow meter is on the inlet side\n    if (Data_Type == 0 || Data_Type == 2) {\n\n       // Find the length of the volume array\n       lenVol = sizeOfDim(outHotGal, 0);\n    //-----------------------------------------------------------------------------------------------\n       /* sum all elements except the last one */\n       if (lenVol > 1) {\n           for (idx = 0; idx < lenVol - 1; idx++) {\n               Gallon += outHotGal[idx];\n           }\n       }\n    //-----------------------------------------------------------------------------------------------\n    }\n//-----------------------------------------------------------------------------------------------\n\n    // This is the case where the flow meter is on the outlet side of the water heater\n    else if (Data_Type == 1) {\n\n       // Find the length of the volume array\n       lenVol = sizeOfDim(outColdGal, 0);\n    //-----------------------------------------------------------------------------------------------\n       /* sum all elements except the last one */\n       if (lenVol > 1) {\n           for (idx = 0; idx < lenVol - 1; idx++) {\n               Gallon += outColdGal[idx];\n           }\n       }\n    //-----------------------------------------------------------------------------------------------\n    }\nTotalGallon      = Gallon ;\n}\n}   // Close the rows >= 1 statement"("Tmin_n_1"=w30, "inColdGal"=w26, "outColdGal"=w26, "inHotGal"=w25, "outHotGal"=w25, "software_time"=w18, "temps"=w17, "hot_total"=w14, "cold_total"=w13, "test_time"=w12, "Data_Type"=w10, "Tavg_deln1"=w9, "Test_Data_Start_End"=w2, "Software_Time_Index"=w1) -> ("Tavg_del_n"=w28:dbl, "Vn"=w29:dbl, "Test_End_Time"=w27:dbl, "outColdGal"=w24:dbl[], "outHotGal"=w23:dbl[], "Factor"=w8:dbl, "Vadd"=w7:dbl, "TotalGallon"=w3:dbl)
  n8 = call "HEWH Get Last Draw Timestamp.vi"("Use Specific Time"=TRUE, "Search Software Elapsed Time"=w27, "error in (no error)"="error in (no error)", "FHD-After 1 hour"=w34, "Test Data-Start to End DBL"=w2) -> ("error out"=→"error out":errorcluster, "Elapsed Time - Last Draw Timestamp"=w32:dbl)  [unwired: 4 in, 1 out]
  n9 = Bundle By Name(cluster="UEF Calculated Values Input", "Calculated Values.Adjustment Factor"=w8, "Calculated Values.Draw Bonus Volume (gal)"=w7, "Sampled Data.Cold Water Draw Amounts-(Gal)"=w24, "Sampled Data.Hot Water Draw Amounts-(Gal)"=w23, "Calculated Values.Vn"=w29, "Calculated Values.T*avg_del(n)"=w28, "Data Indexes.Test End Timestamp"=w27, "Data Indexes.FHD Total Time (Sec)"=w32) -> (w6:T1)
  n10 = case shown="Default" w4 {
    tunnel: w6 -> [w37 w41]
    tunnel: [w38 w40] -> w5
    tunnel: w3 -> [w36 w39]
    frame Default {
      n11 = Bundle By Name(cluster=w37, "Sampled Data.Total Hot Draw Amount (Gal)"=w36) -> (w38:T1)
    }
    frame "GEA Outlet Side Meter" {
      n12 = Bundle By Name(cluster=w41, "Sampled Data.Total Cold Draw Amount (Gal)"=w39) -> (w40:T1)
    }
  }
  "UEF Calculated Values Output" <- w5
